vi "GenerateTestImage.vi"(1 "size":sgl, 2 "ypos":sgl, 3 "xpos":sgl, 4 "tracker":u64) -> (0 "tracker":u64)   [LabVIEW 2011]
uses:
  cudatrack-debug.dll
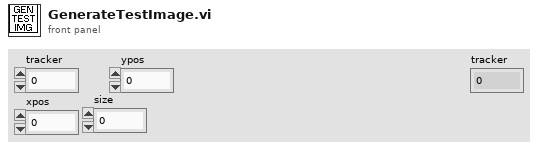
[diagram p1: front panel]
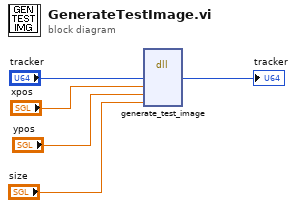
[diagram p0: block diagram]
diagram:
  n1 = dll-call lib="D:/jcnossen1/cudaqi-tracker/cudatrack/cudatrack-debug.dll" fn="generate_test_image"("trackerInstance"="tracker", "xpos"="xpos", "ypos"="ypos", "size"="size") -> ("trackerInstance"=→"tracker":u64)  [unwired: 7 in, 2 out]
